vi "Handle getAll.vi"(8 "error in (no error)":errorcluster, 11 "Instrument.Lockin":refnum<class "Instrument.Lockin.lvclass">) -> (0 "error out":errorcluster, 2 "getAll":variant, 3 "Instrument.Lockin out":refnum<class "Instrument.Lockin.lvclass">)   [LabVIEW 2019, in "Instrument.Lockin.lvclass"]
uses:
  Instrument.Lockin.lvclass
  Instrument.Lockin.lvclass/Instrument.Lockin.ctl
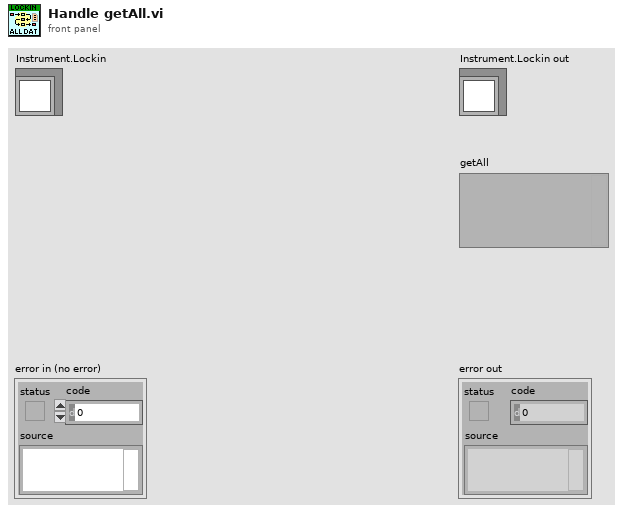
[diagram p1: front panel]
types:
  T1 = typedef "Instrument.Lockin.lvclass/Lockin.getAllData--Cluster.ctl" = cluster{"state":T2, "AO WFM":waveform(dbl)[], "AI WFM":waveform(dbl)[], "REF WFM":waveform(dbl)[], "Results":T3, "SweepWaveforms":T4, "SweepLockinResults":T5}
  T2 = typedef "Lockin.DAQ.lvclass/State-enum.ctl" = enum16{"idle", "created", "started", "stopped", "sweeping"}
  T3 = typedef "Lockin.DAQ.lvclass/Results--Cluster.ctl" = cluster{"Time Stamp":timestamp, "Results (Dictionary)":cluster{"key":string, "value":dbl}[]}
  T4 = typedef "Lockin.DAQ.lvclass/PublicEvents--Lockin.DAQ.getSweepWaveforms.ctl" = cluster{"Sweep_AO":waveform(dbl)[], "Sweep_AI":waveform(dbl)[]}
  T5 = typedef "Lockin.DAQ.lvclass/SweepResults--Cluster.ctl" = cluster{"X results":waveform(dbl)[], "Y Results":waveform(dbl)[]}
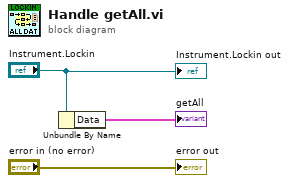
[diagram p0: block diagram]
diagram:
  n1 = Unbundle By Name("Instrument.Lockin") -> ("Data"=→"getAll":T1)
  "error out" <- "error in (no error)"
  "Instrument.Lockin out" <- "Instrument.Lockin"
